vi "Return.vi"() -> ()   [LabVIEW 2016]
uses:
  <vilib>/NXT/Subs/ColorSensorColors.ctl
  <vilib>/NXT/LegoClasses/BrickReference/BrickReference.lvclass
  <vilib>/NXT/Subs/LVHSConnector.ctl
  <vilib>/NXT/Block Support/NXT_InputPort.ctl
panel:
  in  "Port (Port 1)":T1 items=["Port 1", "Port 2", "Port 3", "Port 4"]
  out "NXT/EV3 2":T2
  in  "NXT/EV3":T2
  out "Colors and Directions 2":enum16{"Zero", "Right", "Front", "Left"}[](array[ring])=[enum."Zero", enum."Zero", enum."Zero", enum."Zero", enum."Zero", enum."Zero"]
  in  "Colors and Directions":enum16{"Zero", "Right", "Front", "Left"}[](array[ring])=[enum."Zero", enum."Zero", enum."Zero", enum."Zero", enum."Zero", enum."Zero"]
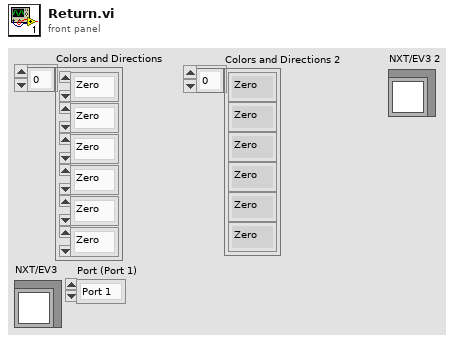
[diagram p1: front panel]
types:
  T1 = typedef "NXT_InputPort.ctl" = u32
  T2 = typedef "LVHSConnector.ctl" = refnum<class "BrickReference.lvclass">
  T3 = typedef "ColorSensorColors.ctl" = enum16{"No Color", "Black", "Blue", "Green", "Yellow", "Red", "White", "Brown"}
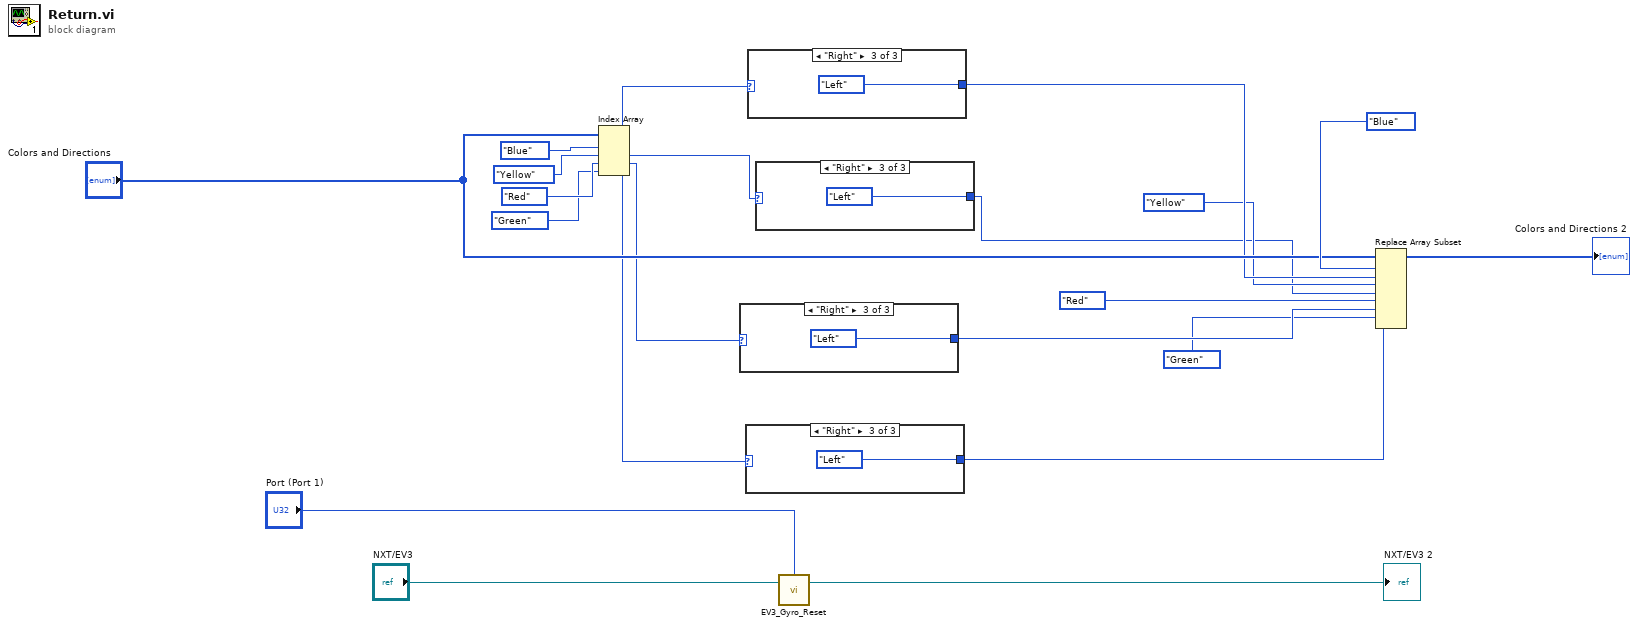
[diagram p0: block diagram]
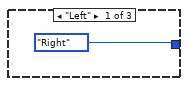
[diagram p2: hidden frame]
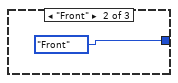
[diagram p3: hidden frame]
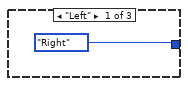
[diagram p4: hidden frame]
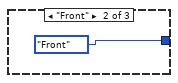
[diagram p5: hidden frame]
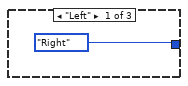
[diagram p6: hidden frame]
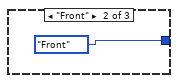
[diagram p7: hidden frame]
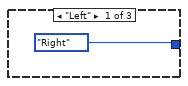
[diagram p8: hidden frame]
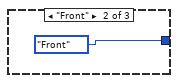
[diagram p9: hidden frame]
diagram:
  n1 = Index Array(array="Colors and Directions", index #1=ColorSensorColors."Blue" ("Detected Color"), index #2=ColorSensorColors."Yellow" ("Detected Color"), index #3=ColorSensorColors."Red" ("Detected Color"), index #4=ColorSensorColors."Green" ("Detected Color")) -> (element #1=w15:enum16{"Zero", "Right", "Front", "Left"}, element #2=w13:enum16{"Zero", "Right", "Front", "Left"}, element #3=w12:enum16{"Zero", "Right", "Front", "Left"}, element #4=w11:enum16{"Zero", "Right", "Front", "Left"})
  n2 = case shown="\"Right\"" w12 {
    tunnel: [enum16{"Zero", "Right", "Front", "Left"}."Right" ("Direction") enum16{"Zero", "Right", "Front", "Left"}."Front" ("Direction") enum16{"Zero", "Right", "Front", "Left"}."Left" ("Direction")] -> w7
    frame "Left" {
    }
    frame "Front" {
    }
    frame "Right" {
    }
  }
  n3 = case shown="\"Right\"" w11 {
    tunnel: [enum16{"Zero", "Right", "Front", "Left"}."Right" ("Direction") enum16{"Zero", "Right", "Front", "Left"}."Front" ("Direction") enum16{"Zero", "Right", "Front", "Left"}."Left" ("Direction")] -> w5
    frame "Left" {
    }
    frame "Front" {
    }
    frame "Right" {
    }
  }
  n4 = case shown="\"Right\"" w15 {
    tunnel: [enum16{"Zero", "Right", "Front", "Left"}."Right" ("Direction") enum16{"Zero", "Right", "Front", "Left"}."Front" ("Direction") enum16{"Zero", "Right", "Front", "Left"}."Left" ("Direction")] -> w14
    frame "Left" {
    }
    frame "Front" {
    }
    frame "Right" {
    }
  }
  n5 = case shown="\"Right\"" w13 {
    tunnel: [enum16{"Zero", "Right", "Front", "Left"}."Right" ("Direction") enum16{"Zero", "Right", "Front", "Left"}."Front" ("Direction") enum16{"Zero", "Right", "Front", "Left"}."Left" ("Direction")] -> w9
    frame "Left" {
    }
    frame "Front" {
    }
    frame "Right" {
    }
  }
  n6 = call <vilib>:"EV3_Gyro_Reset.vi"("NXT/EV3"="NXT/EV3", "Port (Port 1)"="Port (Port 1)") -> ("NXT/EV3"=→"NXT/EV3 2":T2)  [unwired: 2 in]
  n7 = Replace Array Subset(array="Colors and Directions", new element #1=w14, index #1=ColorSensorColors."Blue" ("Detected Color"), new element #2=w9, index #2=ColorSensorColors."Yellow" ("Detected Color"), new element #3=w7, index #3=ColorSensorColors."Red" ("Detected Color"), new element #4=w5, index #4=ColorSensorColors."Green" ("Detected Color")) -> (→"Colors and Directions 2":enum16{"Zero", "Right", "Front", "Left"}[])
